vi "条码补录.vi"() -> ()   [LabVIEW 2018]
uses:
  <vilib>/addons/database/Connection.llb/DB Tools Open Connec (String).vi
  <vilib>/addons/database/NI_Database_API.lvlib
panel:
  in  "选项卡控件":enum32{"条码补录", "产品上线时间补录", "监控"}(tab)
  in  "条 码":string
  in  "确 定":bool
  out "状 态":string
  in  "退 出":bool
  in  "条 码 2":string
  in  "确 定 2":bool
  out "状 态 2":string
  in  "确定按钮":bool
  in  "QRcode":string
  out "数据":string[][](array[string])
  out "数据 2":string[][](array[string])
  out "error out":errorcluster
  # "条码补录（10站）"
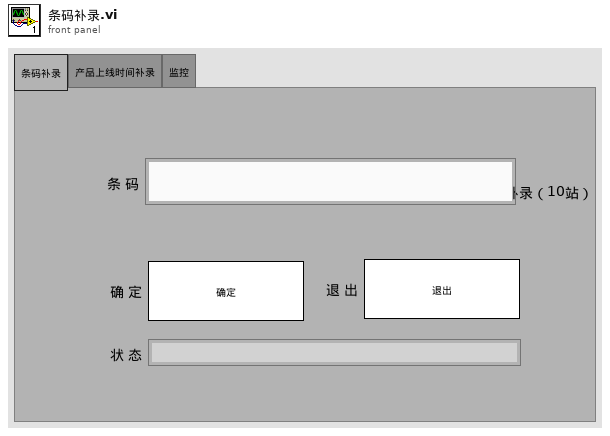
[diagram p1: front panel]
types:
  T1 = typedef "NI_Database_API.lvlib/Conn ObjectReference.ctl" = refnum<k1>
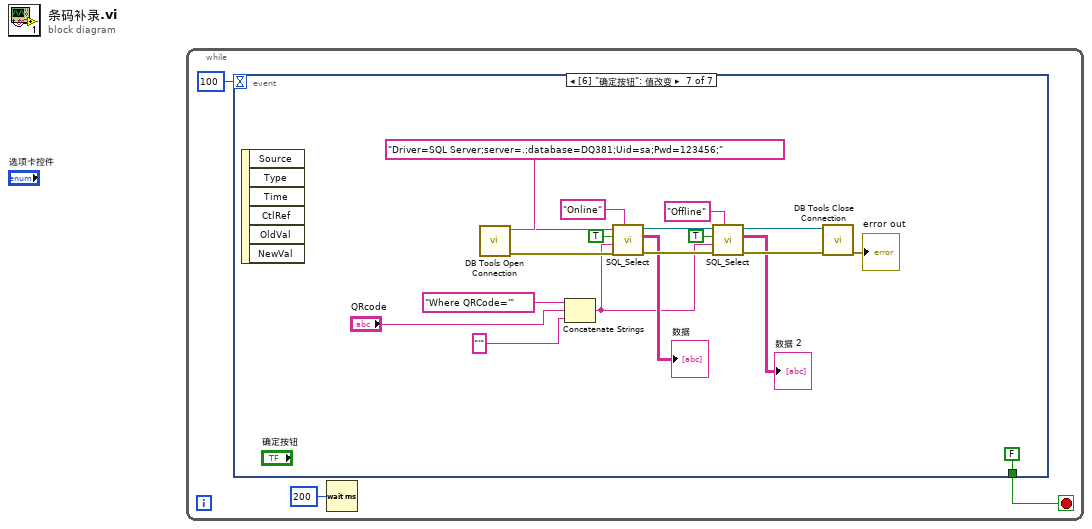
[diagram p0: block diagram]
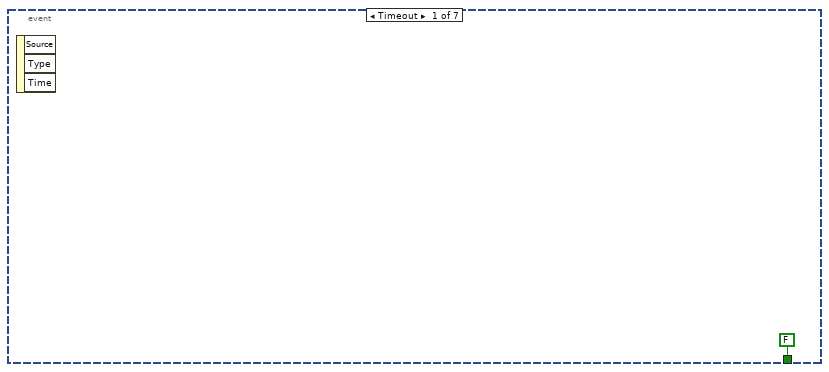
[diagram p2: hidden frame]
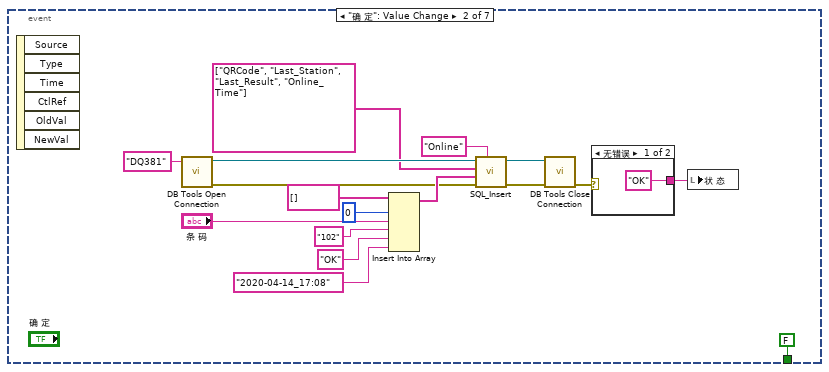
[diagram p3: hidden frame]
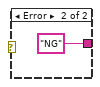
[diagram p4: hidden frame]
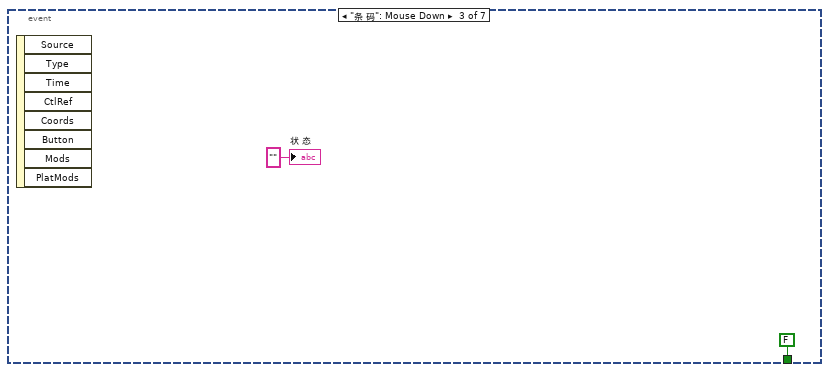
[diagram p5: hidden frame]
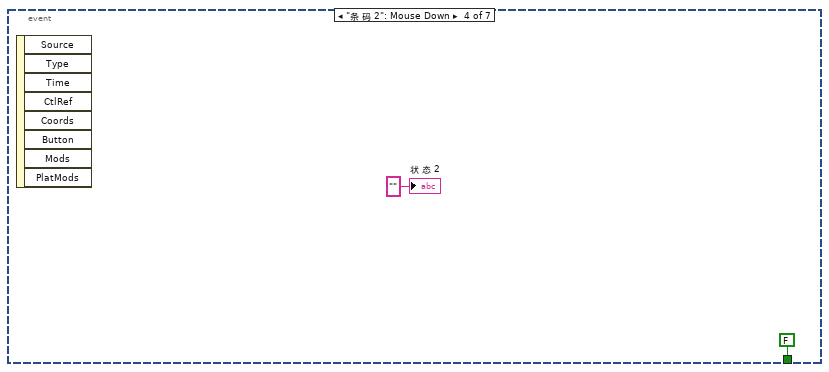
[diagram p6: hidden frame]
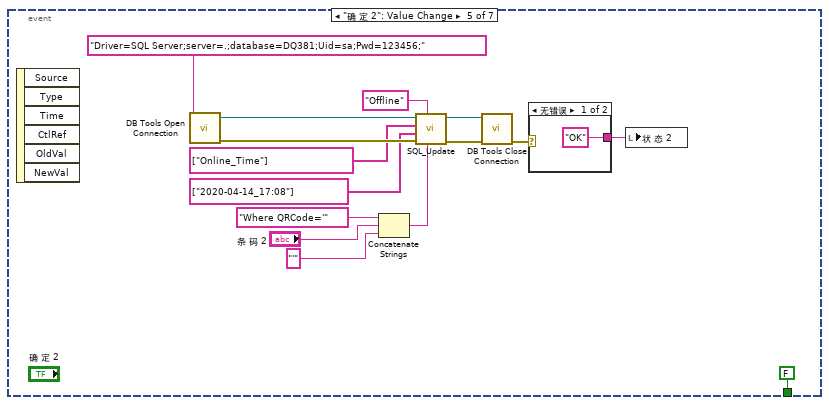
[diagram p7: hidden frame]
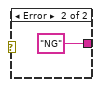
[diagram p8: hidden frame]
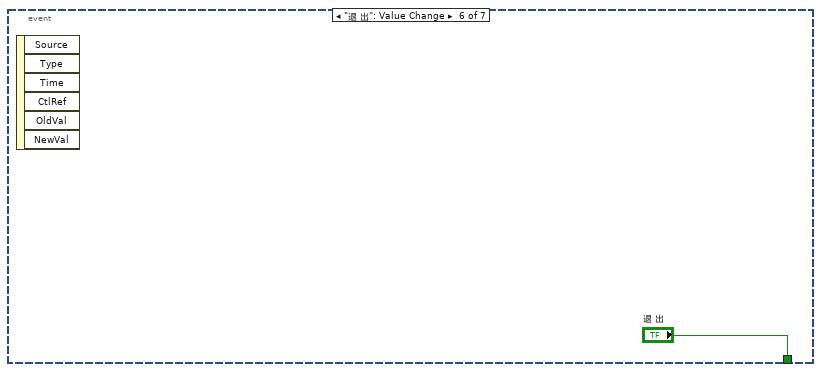
[diagram p9: hidden frame]
diagram:
  n1 = while {
    stop <- w3 stop-if-true
    n2 = event shown="[6] \"确定按钮\": 值改变" {
      selector: _ -> [_ _ _ _ _ _ _]
      dyn-events: _ -> [_ _ _ _ _ _ _]
      timeout: 100 -> [_ _ _ _ _ _ _]
      tunnel: [FALSE ("退 出") FALSE ("退 出") FALSE ("退 出") FALSE ("退 出") FALSE ("退 出") "退 出" FALSE ("退 出")] -> w3
      event Timeout {
        n3 = event-data() -> ()  [unwired: 1 in, 3 out]
      }
      event "确 定": Value Change {
        n4 = event-data() -> ()  [unwired: 1 in, 6 out]
        n5 = call-poly <vilib>:"DB Tools Open Connection.vi"("connection information"="DQ381") -> ("error out"=w20:errorcluster, "connection reference"=w19:T1)  [unwired: 7 in]
        n6 = Insert Into Array(array=string[] [] ("数组"), index=0 ("索引"), new element #1="条 码", new element #2="102" ("新元素/子数组"), new element #3="OK" ("新元素/子数组"), new element #4="2020-04-14_17:08" ("新元素/子数组")) -> (w21:string[])
        n7 = call "SQL_Insert.vi"("表名"="Online", "error in (no error)"=w20, "值"=w21, "列名"=string[] ["QRCode", "Last_Station", "Last_Result", "Online_Time"], "connection reference"=w19) -> ("error out"=w18:errorcluster, "connection reference 2"=w17:T1)  [unwired: 5 in]
        n8 = call <vilib>:"DB Tools Close Connection.vi"("error in (no error)"=w18, "connection reference"=w17) -> ("error out"=w8:errorcluster)  [unwired: 5 in]
        n9 = case shown="无错误" w8 {
          tunnel: ["OK" "NG"] -> w7
          frame No Error {
          }
          frame Error {
          }
        }
        n10 = local write "状 态"(w7) -> ()
      }
      event "条 码": Mouse Down {
        n11 = event-data() -> ()  [unwired: 1 in, 8 out]
        "状 态" <- "" ("状 态")
      }
      event "条 码 2": Mouse Down {
        n12 = event-data() -> ()  [unwired: 1 in, 8 out]
        "状 态 2" <- "" ("状 态 2")
      }
      event "确 定 2": Value Change {
        n13 = event-data() -> ()  [unwired: 1 in, 6 out]
        n14 = call-poly <vilib>:"DB Tools Open Connection.vi"("connection information"="Driver=SQL Server;server=.;database=DQ381;Uid=sa;Pwd=123456;") -> ("error out"=w39:errorcluster, "connection reference"=w40:T1)  [unwired: 7 in]
        n15 = Concatenate Strings("Where QRCode='" ("查询语句"), "条 码 2", "'" ("字符串")) -> (w31:string)
        n16 = call "SQL_Update.vi"("查询语句"=w31, "表名"="Offline", "error in (no error)"=w39, "列名对应的值"=string[] ["2020-04-14_17:08"], "列名"=string[] ["Online_Time"], "connection reference"=w40) -> ("error out"=w35:errorcluster, "connection reference 2"=w34:T1)  [unwired: 4 in]
        n17 = call <vilib>:"DB Tools Close Connection.vi"("error in (no error)"=w35, "connection reference"=w34) -> ("error out"=w36:errorcluster)  [unwired: 5 in]
        n18 = case shown="无错误" w36 {
          tunnel: ["OK" "NG"] -> w28
          frame No Error {
          }
          frame Error {
          }
        }
        n19 = local write "状 态 2"(w28) -> ()
      }
      event "退 出": Value Change {
        n20 = event-data() -> ()  [unwired: 1 in, 6 out]
      }
      event "确定按钮": Value Change {
        n21 = event-data() -> ()  [unwired: 1 in, 6 out]
        n22 = call-poly <vilib>:"DB Tools Open Connection.vi"("connection information"="Driver=SQL Server;server=.;database=DQ381;Uid=sa;Pwd=123456;") -> ("error out"=w55:errorcluster, "connection reference"=w56:T1)  [unwired: 7 in]
        n23 = Concatenate Strings("Where QRCode='" ("查询语句"), "QRcode", "'" ("字符串")) -> (w48:string)
        n24 = call "SQL_Select.vi"("表名"="Online", "error in (no error)"=w55, "查询语句"=w48, "查询条件"=TRUE, "connection reference"=w56) -> ("error out"=w60:errorcluster, "数据"=→"数据":string[][], "connection reference out"=w59:T1)  [unwired: 4 in]
        n25 = call "SQL_Select.vi"("表名"="Offline", "error in (no error)"=w60, "查询语句"=w48, "查询条件"=TRUE, "connection reference"=w59) -> ("error out"=w54:errorcluster, "数据"=→"数据 2":string[][], "connection reference out"=w53:T1)  [unwired: 4 in]
        n26 = call <vilib>:"DB Tools Close Connection.vi"("error in (no error)"=w54, "connection reference"=w53) -> ("error out"=→"error out":errorcluster)  [unwired: 5 in]
      }
    }
    n27 = Wait (ms)(milliseconds to wait=u32 200 ("等待时间（毫秒）")) -> ()  [unwired: 1 out]
  }
